vi "TAT_Communication setting Read.vi"(8 "error in (no error)":errorcluster) -> (0 "error out":errorcluster, 1 "PLC IP":string, 2 "Ass Scanner Port":string, 3 "Torque Scanner Port":string, 4 "Printer Port":u32, 5 "Screw Driver Port":u32, 6 "Printer IP":string="com1", 7 "Screw Driver IP":string)   [LabVIEW 2017]
uses:
  <vilib>/Utility/config.llb/Read Key (String).vi
  <vilib>/Utility/config.llb/Read Key (U32).vi
  <vilib>/Utility/config.llb/NI_LVConfig.lvlib
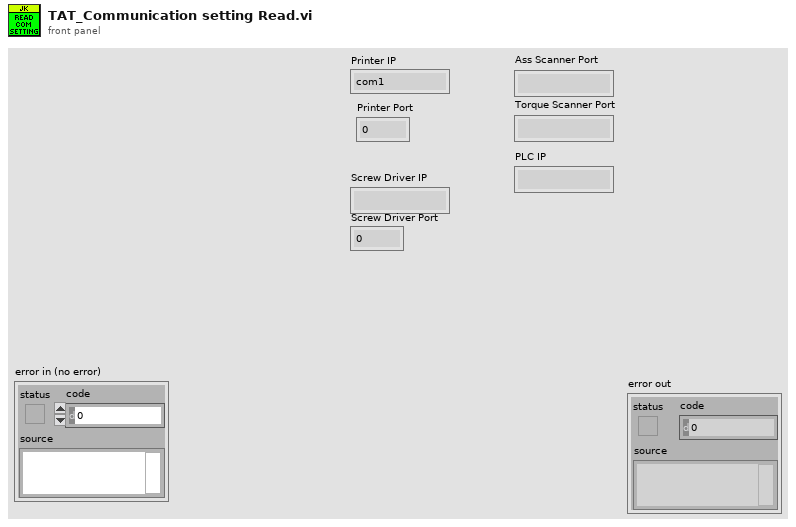
[diagram p1: front panel]
types:
  T1 = enum32{"invalid app kind", "Development System", "Run Time System", "Student Edition", "Embedded LabVIEW", "Evaluation", "Custom"}
  T2 = typedef "NI_LVConfig.lvlib/Config Data RefNum.ctl" = refnum<k1>
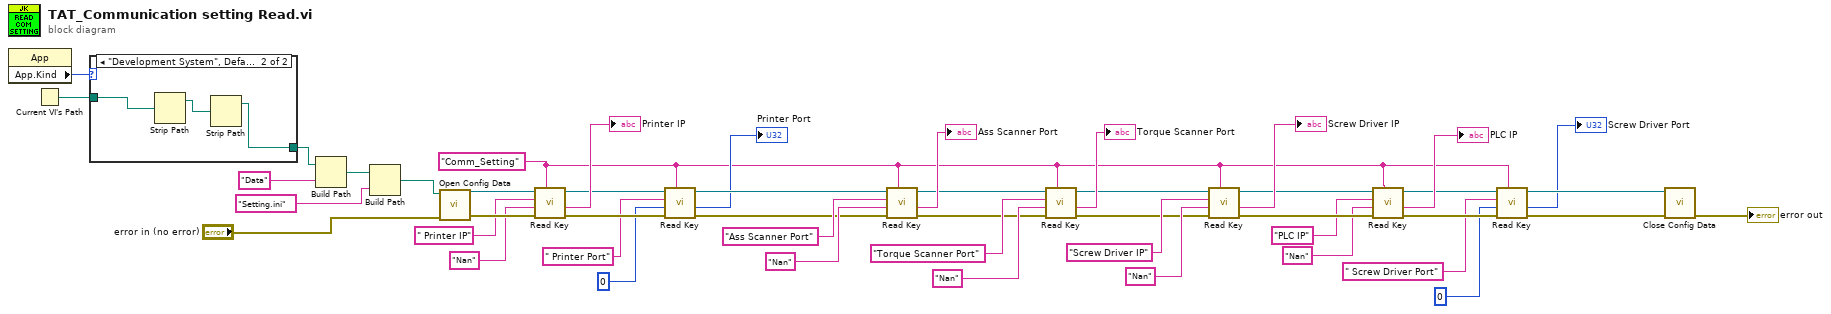
[diagram p0: block diagram]
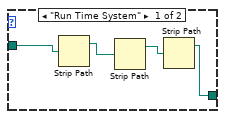
[diagram p2: hidden frame]
diagram:
  w3 = "Comm_Setting" ("section")
  n1 = property class="App"() -> ("App.Kind"=w46:T1)  [unwired: 2 in, 2 out]
  n2 = Current VI's Path() -> (path=w47:path)
  n3 = case shown="\"Development System\", Default" w46 {
    tunnel: w47 -> [w49 w53]
    tunnel: [w48 w52] -> w44
    frame "Run Time System" {
      n4 = Strip Path(path=w49) -> (stripped path=w51:path)  [unwired: 1 out]
      n5 = Strip Path(path=w51) -> (stripped path=w50:path)  [unwired: 1 out]
      n6 = Strip Path(path=w50) -> (stripped path=w48:path)  [unwired: 1 out]
    }
    frame "Development System", Default {
      n7 = Strip Path(path=w53) -> (stripped path=w54:path)  [unwired: 1 out]
      n8 = Strip Path(path=w54) -> (stripped path=w52:path)  [unwired: 1 out]
    }
  }
  n9 = Build Path(base path=w44, name or relative path="Data") -> (appended path=w45:path)
  n10 = Build Path(base path=w45, name or relative path="Setting.ini") -> (appended path=w41:path)
  n11 = call <vilib>:"Open Config Data.vi"("error in (no error)"="error in (no error)", "configuration file path"=w41) -> ("error out"=w39:errorcluster, "refnum"=w38:T2)  [unwired: 7 in, 1 out]
  n12 = call-poly <vilib>:"Read Key.vi"("section"=w3, "error in (no error)"=w39, "default value"="Nan", "key"=" Printer IP", "refnum"=w38) -> ("error out"=w13:errorcluster, "value"=→"Printer IP":string, "refnum out"=w15:T2)  [unwired: 3 in, 1 out]
  n13 = call-poly <vilib>:"Read Key.vi"("section"=w3, "error in (no error)"=w13, "default value"=u32 0, "key"=" Printer Port", "refnum"=w15) -> ("error out"=w12:errorcluster, "value"=→"Printer Port":u32, "refnum out"=w14:T2)  [unwired: 3 in, 1 out]
  n14 = call-poly <vilib>:"Read Key.vi"("section"=w3, "error in (no error)"=w12, "default value"="Nan", "key"="Ass Scanner Port", "refnum"=w14) -> ("error out"=w18:errorcluster, "value"=→"Ass Scanner Port":string, "refnum out"=w19:T2)  [unwired: 3 in, 1 out]
  n15 = call-poly <vilib>:"Read Key.vi"("section"=w3, "error in (no error)"=w18, "default value"="Nan", "key"="Torque Scanner Port", "refnum"=w19) -> ("error out"=w17:errorcluster, "value"=→"Torque Scanner Port":string, "refnum out"=w16:T2)  [unwired: 3 in, 1 out]
  n16 = call-poly <vilib>:"Read Key.vi"("section"=w3, "error in (no error)"=w17, "default value"="Nan", "key"="Screw Driver IP", "refnum"=w16) -> ("error out"=w26:errorcluster, "value"=→"Screw Driver IP":string, "refnum out"=w27:T2)  [unwired: 3 in, 1 out]
  n17 = call-poly <vilib>:"Read Key.vi"("section"=w3, "error in (no error)"=w26, "default value"="Nan", "key"="PLC IP", "refnum"=w27) -> ("error out"=w6:errorcluster, "value"=→"PLC IP":string, "refnum out"=w8:T2)  [unwired: 3 in, 1 out]
  n18 = call-poly <vilib>:"Read Key.vi"("section"=w3, "error in (no error)"=w6, "default value"=u32 0, "key"=" Screw Driver Port", "refnum"=w8) -> ("error out"=w5:errorcluster, "value"=→"Screw Driver Port":u32, "refnum out"=w7:T2)  [unwired: 3 in, 1 out]
  n19 = call <vilib>:"Close Config Data.vi"("error in (no error)"=w5, "refnum"=w7) -> ("error out"=→"error out":errorcluster)  [unwired: 8 in, 1 out]
